vi "Actor Core.vi"(8 "error in":errorcluster, 11 "GObject View in":refnum<class "Resource View.lvclass">) -> (0 "error out":errorcluster, 3 "Actor out":refnum<class "Actor.lvclass">)   [LabVIEW 2013, in "SET Project Editor.lvlib" / "Resource View.lvclass"]
doc: "(<B>Filename</B>: Actor Framework.lvlib:Actor.lvclass:Actor Core.vi)\n\nReceives messages to the actor, reacts to them, and initiates any error handling that may shut the actor down.\n\nDescendant classes may override this VI to append parallel tasks for the actor to complete while it handles messages. Overrides use the Call Parent Method node."
uses:
  Resource View.lvclass
  <vilib>/ActorFramework/Actor/Actor.lvclass
  <vilib>/Utility/miscctls.llb/LVRowAndColumnTypeDef.ctl
  <vilib>/ActorFramework/Actor/Actor.lvclass/Actor.ctl
  <vilib>/ActorFramework/Message Enqueuer/Message Enqueuer.lvclass/Message Enqueuer.ctl
  Controller Messages/Remove Shared Resource Msg/Remove Shared Resource Msg.lvclass/Remove Shared Resource Msg.ctl
  Controller Messages/Edit Shared Resource Msg/Edit Shared Resource Msg.lvclass/Edit Shared Resource Msg.ctl
  MCListbox View Messages/MCLB Request Edit Cell Msg/MCLB Request Edit Cell Msg.lvclass/MCLB Request Edit Cell Msg.ctl
  MCListbox View/MCListbox View.lvclass/MCListbox View.ctl
  MCListbox View/MCListbox View.lvclass
  MCListbox View/Properties/Write Editable From.vi
  <vilib>/ActorFramework/Message Enqueuer/Init from Existing Queue.vi
  <vilib>/ActorFramework/Message Enqueuer/Enqueue.vi
  <vilib>/ActorFramework/Message Priority Queue/Priority Enqueue.vi
  <vilib>/ActorFramework/Message Enqueuer/Message Enqueuer.lvclass
  <vilib>/ActorFramework/Stop Msg/Stop Msg.lvclass
  Controller Messages/Remove Shared Resource Msg/Remove Shared Resource Msg.lvclass
  Controller Messages/Edit Shared Resource Msg/Edit Shared Resource Msg.lvclass
  Controller Messages/Add Shared Resource Msg/Add Shared Resource Msg.lvclass
  MCListbox View Messages/MCLB Request Edit Cell Msg/MCLB Request Edit Cell Msg.lvclass
  MCListbox View Messages/MCLB StrEdit Resize Msg/MCLB StrEdit Resize Msg.lvclass
  Lib/Unicode/SET_Unicode Tools.lvlib
panel:
  in  "StrEdit":string
  in  "Items":i32(listbox)
  # "Shared Resources"
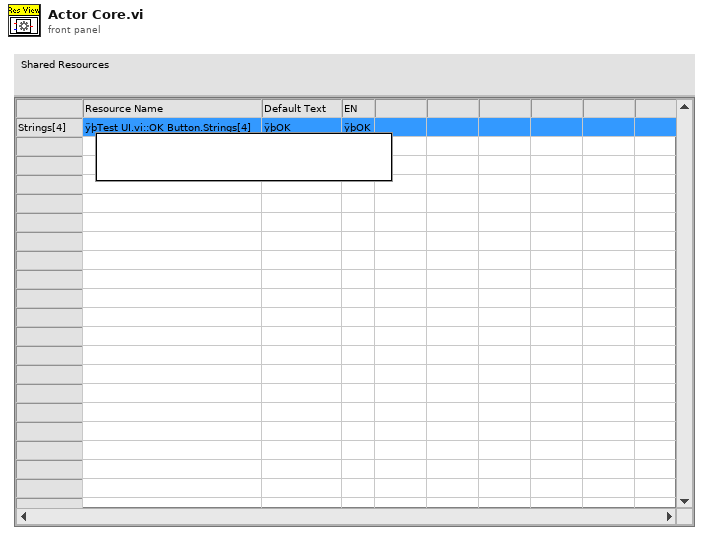
[diagram p1: front panel]
types:
  T1 = typedef "LVRowAndColumnTypeDef.ctl" = cluster{"Row":i32, "Column":i32}
  T2 = typedef "LVPoint32TypeDef.ctl" = cluster{"Horizontal":i32, "Vertical":i32}
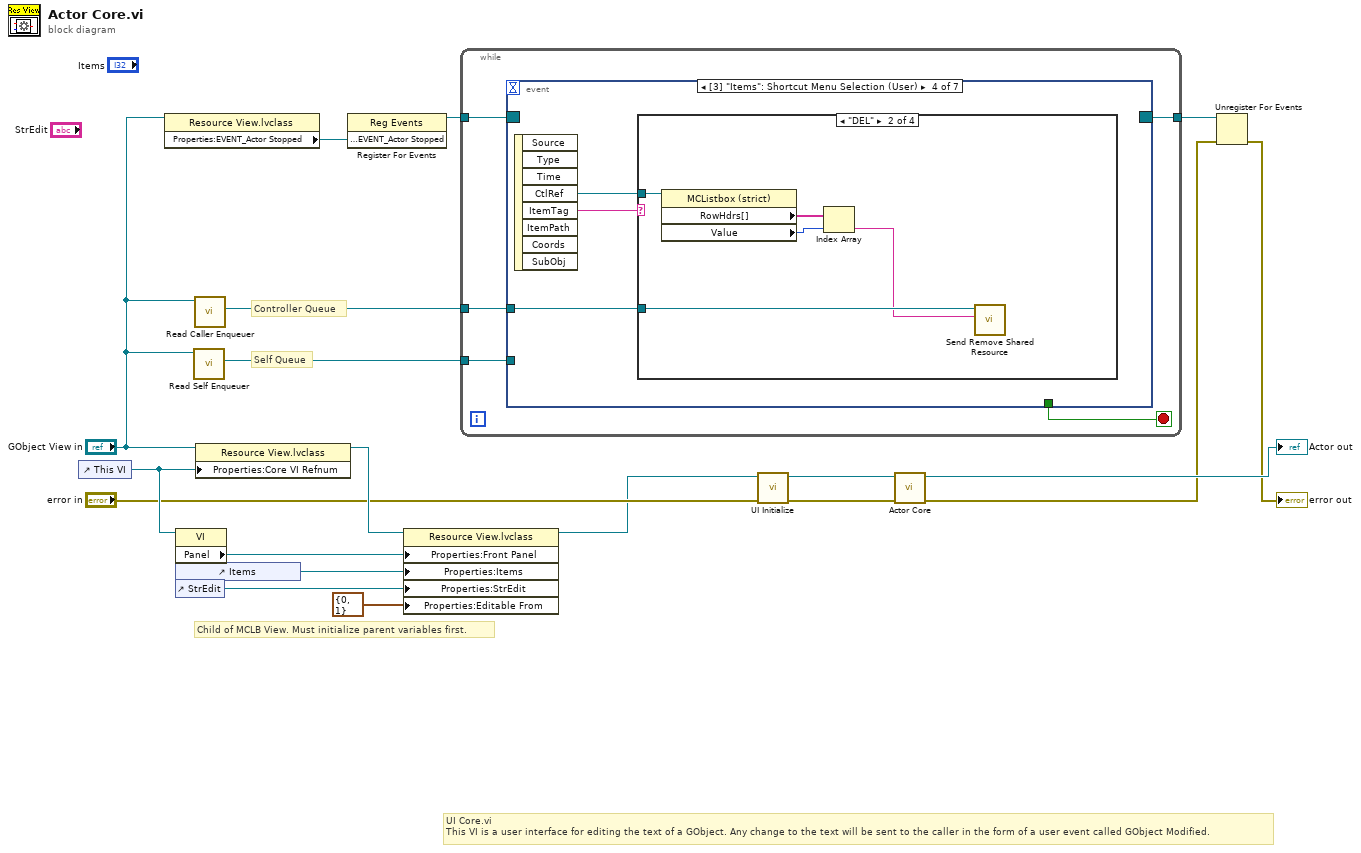
[diagram p0: block diagram]
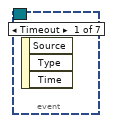
[diagram p2: hidden frame]
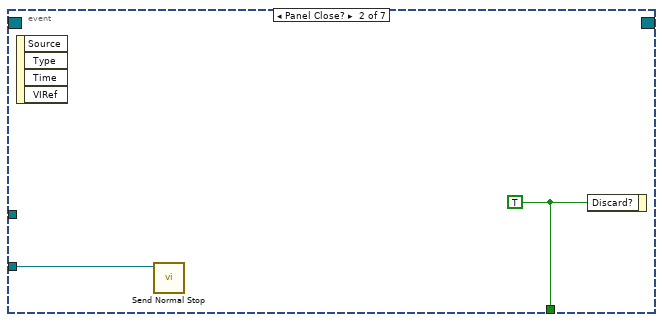
[diagram p3: hidden frame]
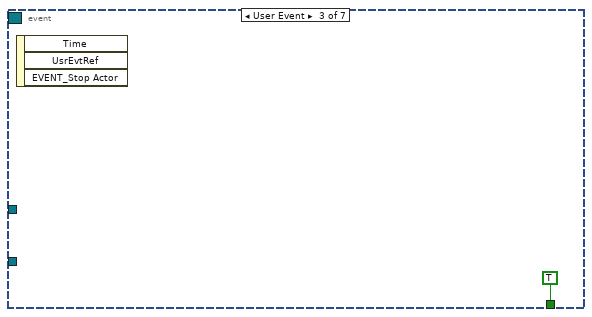
[diagram p4: hidden frame]
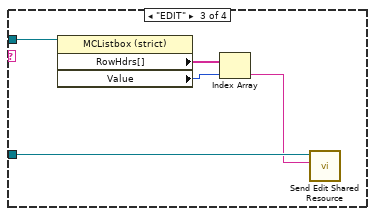
[diagram p6: hidden frame]
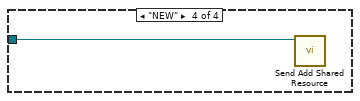
[diagram p7: hidden frame]
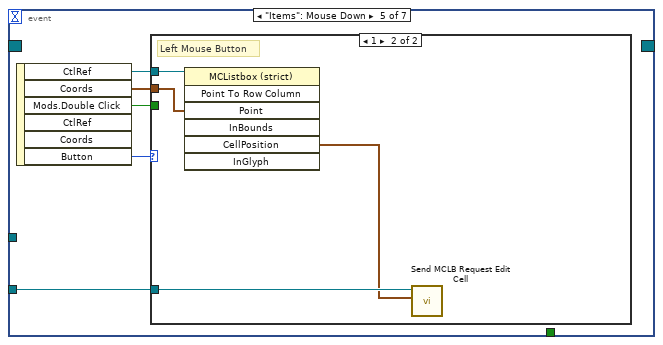
[diagram p8: hidden frame]
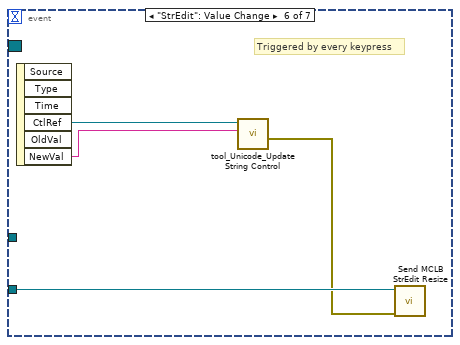
[diagram p10: hidden frame]
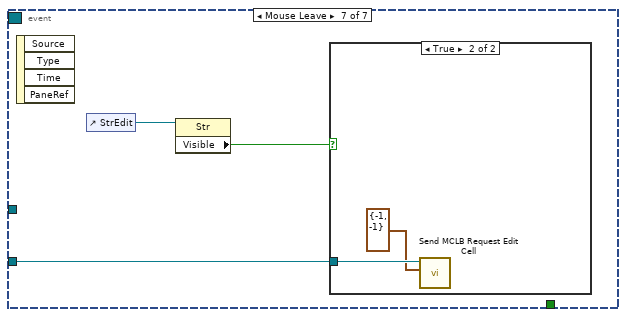
[diagram p11: hidden frame]
diagram:
  # "Child of MCLB View. Must initialize parent variables first."
  # "Controller Queue"
  # "UI Core.vi\nThis VI is a user interface for editing the text of a GObject. Any change to the text will be sent to the caller in the form of a user event called GObject Modified."
  # "Self Queue"
  n1 = control-ref of="This VI"() -> (w11:refnum<vi>)
  n2 = property class="Resource View.lvclass"(reference="GObject View in") -> ("Properties:EVENT_Actor Stopped"=w18:refnum<user-event>)  [unwired: 1 in, 2 out]
  n3 = property class="VI"(reference=w11) -> ("Panel"=w8:refnum<vi>)  [unwired: 1 in, 2 out]
  n4 = control-ref of="Items"() -> (w7:refnum<vi>)
  n5 = control-ref of="StrEdit"() -> (w6:refnum<vi>)
  n6 = call <vilib>:"Read Self Enqueuer.vi"("Actor"="GObject View in") -> ("Self Enqueuer"=w10:refnum<class "Message Enqueuer.lvclass">)  [unwired: 10 in]
  n7 = call <vilib>:"Read Caller Enqueuer.vi"("Actor"="GObject View in") -> ("Caller Enqueuer"=w13:refnum<class "Message Enqueuer.lvclass">)  [unwired: 10 in]
  n8 = property class="Resource View.lvclass"(reference="GObject View in", "Properties:Core VI Refnum"=w11) -> (reference out=w9:refnum<class "Resource View.lvclass">)  [unwired: 1 in, 1 out]
  n9 = register-events(w18) -> (reference out=w17:refnum<event-registration>)  [unwired: 2 in, 1 out]
  n10 = property class="Resource View.lvclass"(reference=w9, "Properties:Front Panel"=w8, "Properties:Items"=w7, "Properties:StrEdit"=w6, "Properties:Editable From"=T1 {"Row"=0, "Column"=1} ("Editable From")) -> (reference out=w1:refnum<class "Resource View.lvclass">)  [unwired: 1 in, 1 out]
  n11 = while {
    tunnel: w17 -> [w23]
    tunnel: [w22] -> w16
    tunnel: w10 -> [w21]
    tunnel: w13 -> [w20]
    stop <- w24 stop-if-true
    n12 = event shown="[3] \"Items\": Shortcut Menu Selection (User)" {
      selector: w23 -> [_ _ _ _ _ _ _]
      dyn-events: [_ _ _ _ _ _ _] -> w22
      timeout: _ -> [_ _ _ _ _ _ _]
      tunnel: [_ w26 TRUE ("Discard?") _ _ _ _] -> w24
      tunnel: w21 -> [_ w25 _ _ w42 w52 w55]
      tunnel: w20 -> [_ _ _ w28 _ _ _]
      event Timeout {
        n13 = event-data() -> ()  [unwired: 1 in, 3 out]
      }
      event Panel Close? {
        w26 = TRUE ("Discard?")
        n14 = event-data() -> ()  [unwired: 1 in, 4 out]
        n15 = call <vilib>:"Send Normal Stop.vi"("Message Enqueuer"=w25) -> ()  [unwired: 10 in, 1 out]
        n16 = event-data("Discard?"=w26) -> ()  [unwired: 1 in, 1 out]
      }
      event User Event {
        n17 = event-data() -> ()  [unwired: 1 in, 3 out]
      }
      event "Items": Shortcut Menu Selection (User) {
        n18 = event-data() -> ("CtlRef"=w29:refnum<vi>, "ItemTag"=w30:string)  [unwired: 1 in, 6 out]
        n19 = case shown="\"DEL\"" w30 {
          tunnel: w29 -> [_ w32 w40 _]
          tunnel: w28 -> [_ w35 w37 w41]
          frame Default {
          }
          frame "DEL" {
            n20 = property class="MCListbox (strict)"(reference=w32) -> ("RowHdrs[]"=w34:string[], "Value"=w33:i32)  [unwired: 1 in, 2 out]
            n21 = Index Array(array=w34, index=w33) -> (element=w31:string)
            n22 = call "Send Remove Shared Resource.vi"("RID"=w31, "Message Enqueuer"=w35) -> ()  [unwired: 8 in, 2 out]
          }
          frame "EDIT" {
            n23 = property class="MCListbox (strict)"(reference=w40) -> ("RowHdrs[]"=w39:string[], "Value"=w38:i32)  [unwired: 1 in, 2 out]
            n24 = Index Array(array=w39, index=w38) -> (element=w36:string)
            n25 = call "Send Edit Shared Resource.vi"("RID"=w36, "Message Enqueuer"=w37) -> ()  [unwired: 8 in, 2 out]
          }
          frame "NEW" {
            n26 = call "Send Add Shared Resource.vi"("Message Enqueuer"=w41) -> ()  [unwired: 9 in, 2 out]
          }
        }
      }
      event "Items": Mouse Down {
        n27 = event-data() -> ("CtlRef"=w45:refnum<vi>, "Coords"=w44:T2, "Mods.Double Click"=w43:bool, "Button"=w46:u16)  [unwired: 1 in, 2 out]
        n28 = case shown="1" w46 {
          tunnel: w45 -> [_ w50]
          tunnel: w44 -> [_ w49]
          tunnel: w43 -> [_ _]
          tunnel: w42 -> [_ w48]
          frame 0, Default {
          }
          frame 1 {
            # "Left Mouse Button"
            n29 = invoke class="MCListbox (strict)" method="Point To Row Column"(reference=w50, "Point"=w49) -> ("CellPosition"=w47:T1)  [unwired: 5 in, 6 out]
            n30 = call "Send MCLB Request Edit Cell.vi"("RowAndCollumn"=w47, "Message Enqueuer"=w48) -> ()  [unwired: 8 in, 2 out]
          }
        }
      }
      event "StrEdit": Value Change {
        # "Triggered by every keypress"
        n31 = event-data() -> ("CtlRef"=w54:refnum<vi>, "NewVal"=w53:string)  [unwired: 1 in, 4 out]
        n32 = call "tool_Unicode_Update String Control.vi"("String (UTF-16)"=w53, "*StrControl in"=w54) -> ("error out"=w51:errorcluster)  [unwired: 8 in, 1 out]
        n33 = call "Send MCLB StrEdit Resize.vi"("error in (no error)"=w51, "Message Enqueuer"=w52) -> ()  [unwired: 8 in, 2 out]
      }
      event Mouse Leave {
        n34 = event-data() -> ()  [unwired: 1 in, 4 out]
        n35 = control-ref of="StrEdit"() -> (w57:refnum<vi>)
        n36 = property class="Str"(reference=w57) -> ("Visible"=w56:bool)  [unwired: 1 in, 2 out]
        n37 = case shown="True" w56 {
          tunnel: w55 -> [_ w59]
          frame False {
          }
          frame True {
            n38 = call "Send MCLB Request Edit Cell.vi"("RowAndCollumn"=T1 {"Row"=-1, "Column"=-1} ("Cell Position"), "Message Enqueuer"=w59) -> ()  [unwired: 8 in, 2 out]
          }
        }
      }
    }
  }
  n39 = call-dynamic "UI Initialize.vi"("error in (no error)"="error in", "GObject View in"=w1) -> ("error out"=w3:errorcluster, "GObject View out"=w4:refnum<class "Resource View.lvclass">)  [unwired: 8 in]
  n40 = call-parent "Actor Core.vi"("error in"=w3, "Actor in"=w4) -> ("error out"=w15:errorcluster, "Actor out"=→"Actor out":refnum<class "Actor.lvclass">)  [unwired: 8 in]
  n41 = Unregister For Events(event registration refnum=w16, error in=w15) -> (error out=→"error out":errorcluster)
